vi "Smart IO Configure LED Device.vi"(8 "error in (no error)":errorcluster, 9 "length":i32, 10 "startIndex":i32, 11 "deviceIndex":i32) -> (0 "error out":errorcluster, 3 "deviceIndex out":i32)   [LabVIEW 2026, in "MrcLib.lvlib"]
doc: "Update the LED start/length span configuration for the wired device channel. Spans of different device channels can overlap to share LED buffer colors, and a negative length can be used if you want to share, but in reverse order."
uses:
  MrcLib.lvlib
  Types/MRC Smart IO Mode.ctl
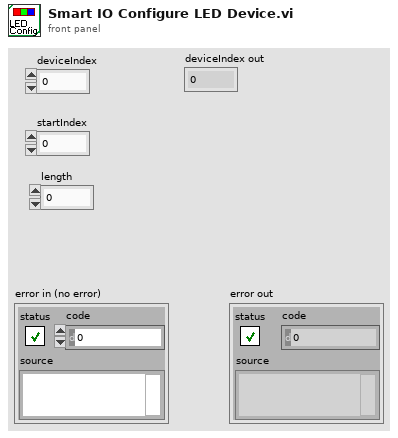
[diagram p1: front panel]
types:
  T1 = typedef "MRC Smart IO Mode.ctl" = i32
  T2 = enum16{"update device span", "update LED buffer", "clear"}
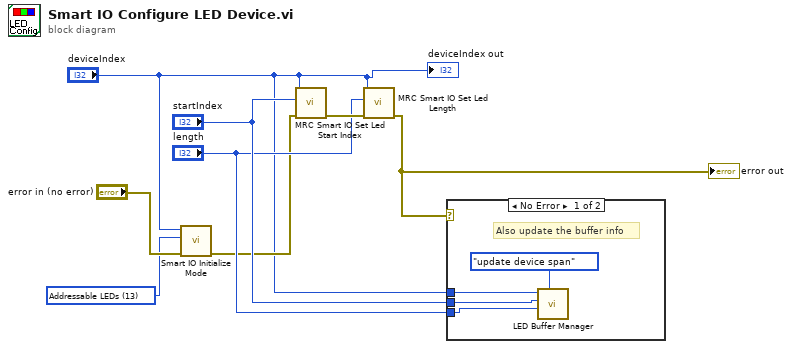
[diagram p0: block diagram]
diagram:
  w1 = T1 13 items=["Digital Input"=0, "Digital Output"=1, "Analog Input"=2, "PWM Input"=3, "PWM Output"=4, "Counter Rising"=5, "Counter Falling"=6, "Addressable LEDs"=13] ("mode")
  n1 = call "Smart IO Initialize Mode.vi"("error in (no error)"="error in (no error)", "mode"=w1, "deviceIndex"="deviceIndex") -> ("error out"=w3:errorcluster)  [unwired: 8 in]
  n2 = call "MRC Smart IO Set Led Start Index.vi"("error in (no error)"=w3, "startIndex"="startIndex", "deviceIndex"="deviceIndex") -> ("error out"=w8:errorcluster)  [unwired: 8 in]
  n3 = call "MRC Smart IO Set Led Length.vi"("error in (no error)"=w8, "length"="length", "deviceIndex"="deviceIndex") -> ("error out"=w7:errorcluster)  [unwired: 8 in]
  "error out" <- w7
  n4 = case shown="No Error" w7 {
    tunnel: "deviceIndex" -> [w12 _]
    tunnel: "startIndex" -> [w11 _]
    tunnel: "length" -> [w10 _]
    frame No Error {
      # "Also update the buffer info"
      n5 = call "LED Buffer Manager.vi"("action"=T2."update device span", "length"=w10, "startIndex"=w11, "deviceIndex"=w12) -> ()  [unwired: 8 in]
    }
    frame Error {
    }
  }
  "deviceIndex out" <- "deviceIndex"
